vi "DurationTime.vi"(8 "error in":errorcluster, 11 "Starttime (Ticks in ms)":u32) -> (0 "error out":errorcluster, 3 "Time (ms)":u32)   [LabVIEW 2015]
panel:
  # "Input: Starting time\n\nOutput: Difference between Starting time and \nthe time this block is called.\n\nUse the Error-Line to call this block after your \nprogram-algorithm"
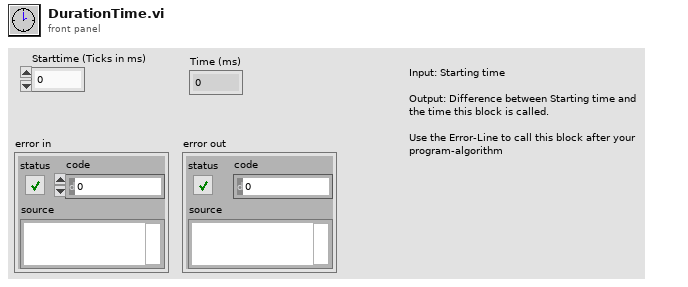
[diagram p1: front panel]
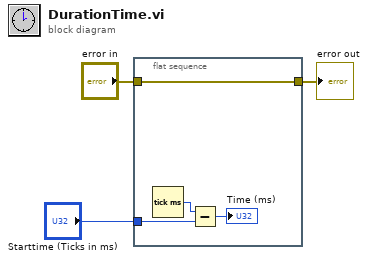
[diagram p0: block diagram]
diagram:
  n1 = flat-sequence {
    tunnel: "Starttime (Ticks in ms)" -> [w6]
    tunnel: [w4] -> w1
    tunnel: "error in" -> [w4]
    frame #0 {
      n2 = Tick Count (ms)() -> (millisecond timer value=w7:u32)
      n3 = Subtract(x=w7, y=w6) -> (x-y=→"Time (ms)":u32)
    }
  }
  "error out" <- w1
